vi "CFTS-Parse Folder Name.vi"(0 "Path":path) -> (4 "User ID":string, 6 "Animal ID":i32, 10 "Exists?":bool)   [LabVIEW 2020]
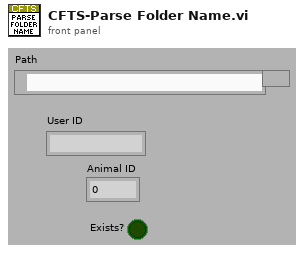
[diagram p1: front panel]
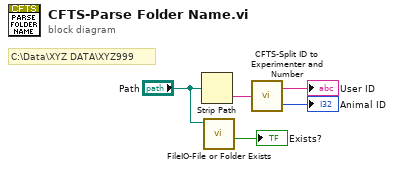
[diagram p0: block diagram]
diagram:
  # "C:\\Data\\XYZ DATA\\XYZ999"
  n1 = Strip Path(path="Path") -> (name=w3:string)  [unwired: 1 out]
  n2 = call "FileIO-File or Folder Exists.vi"("path"="Path") -> ("Exists?"=→"Exists?":bool)  [unwired: 7 in, 3 out]
  n3 = call "CFTS-Split ID to Experimenter and Number.vi"("ID"=w3) -> ("Experimenter"=→"User ID":string, "Number"=→"Animal ID":i32)
